vi "BlackJack21.vi"() -> ()   [LabVIEW 2019]
panel:
  out "DRAW":bool
  out "LOSE":bool
  in  "BUST":bool
  out "WIN":bool
  out "DealerCard#5":u16(ring)
  out "CP-Dealer#5":dbl
  out "DealerCard#4":u16(ring)
  out "CP-Dealer#4":dbl
  in  "STAND POS":dbl
  out "SAME CARD DETECTED":bool
  out "DealerCard#3":u16(ring)
  out "CP-Dealer#3":dbl
  out "UserCard#5":u16(ring)
  out "CP-User#5":dbl
  in  "HIT POS":i32
  out "UserCard#4":u16(ring)
  out "CP-User#4":dbl
  out "DealerCard#2":u16(ring)
  out "CP-Dealer#2":dbl
  out "Total Player Point":dbl
  out "Total Dealer Point":dbl
  out "DealerCard#1":u16(ring)
  out "CP-Dealer#1":dbl
  out "UserCard#3":u16(ring)
  out "CP-User#3":dbl
  out "UserCard#2":u16(ring)
  out "CP-User#2":dbl
  in  "RESTART GAME":bool
  in  "STAND":bool
  out "Numeric":i32
  in  "EMERGENCY STOP":bool
  in  "START GAME":bool
  out "CP-User#1":dbl
  out "UserCard#1":u16(ring)
  in  "Hit":bool
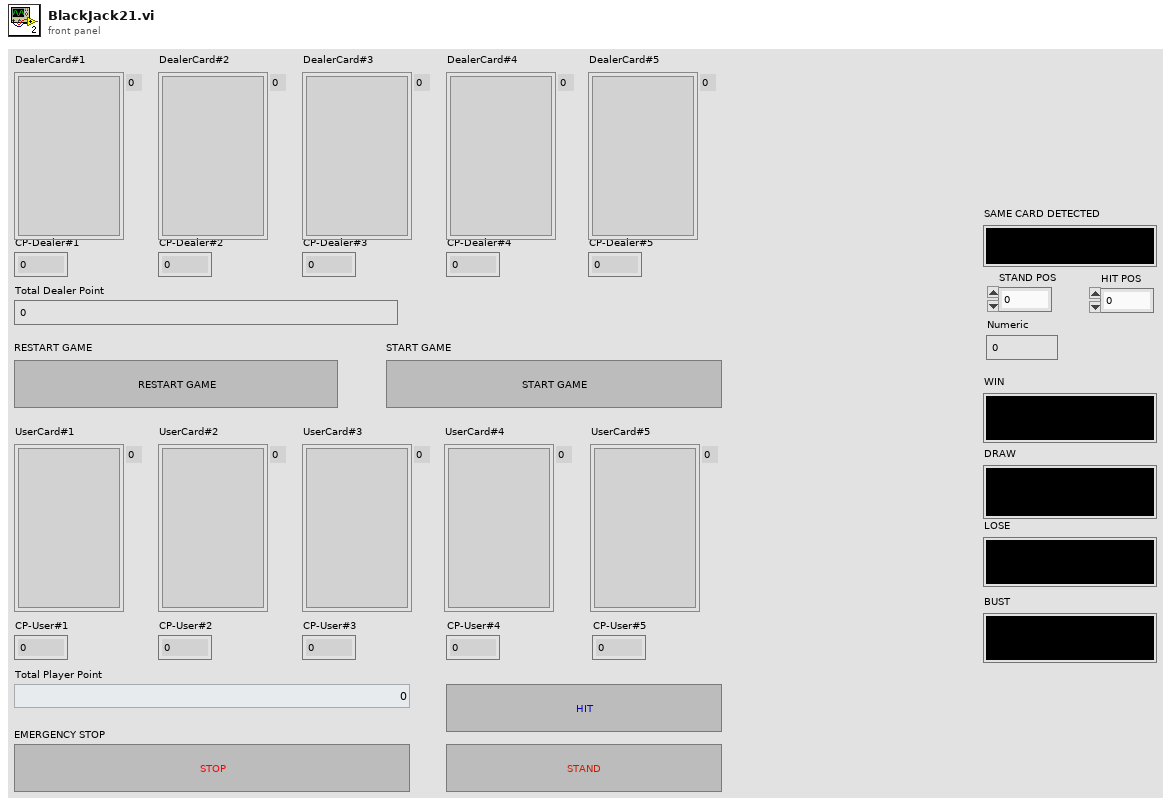
[diagram p1: front panel]
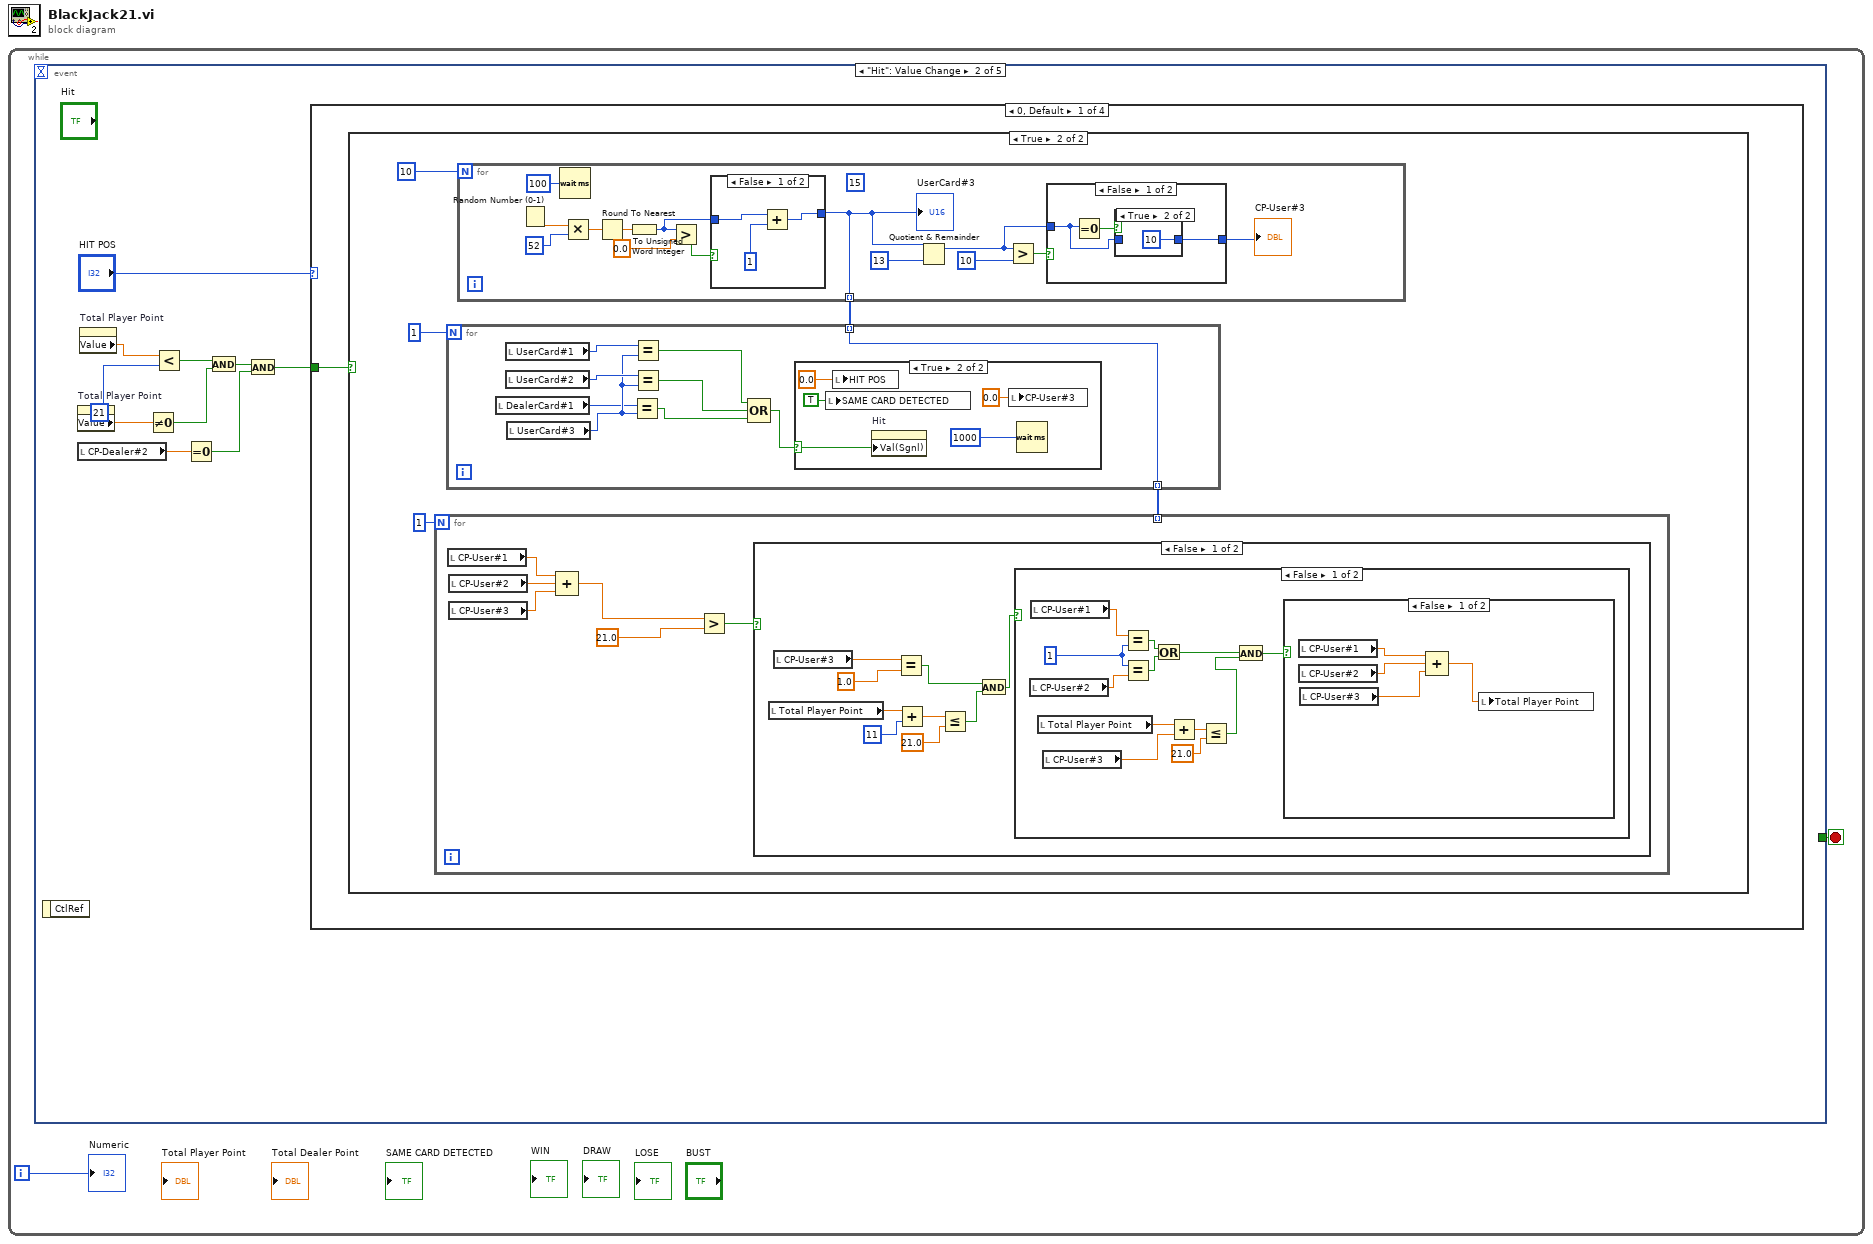
[diagram p0: block diagram]
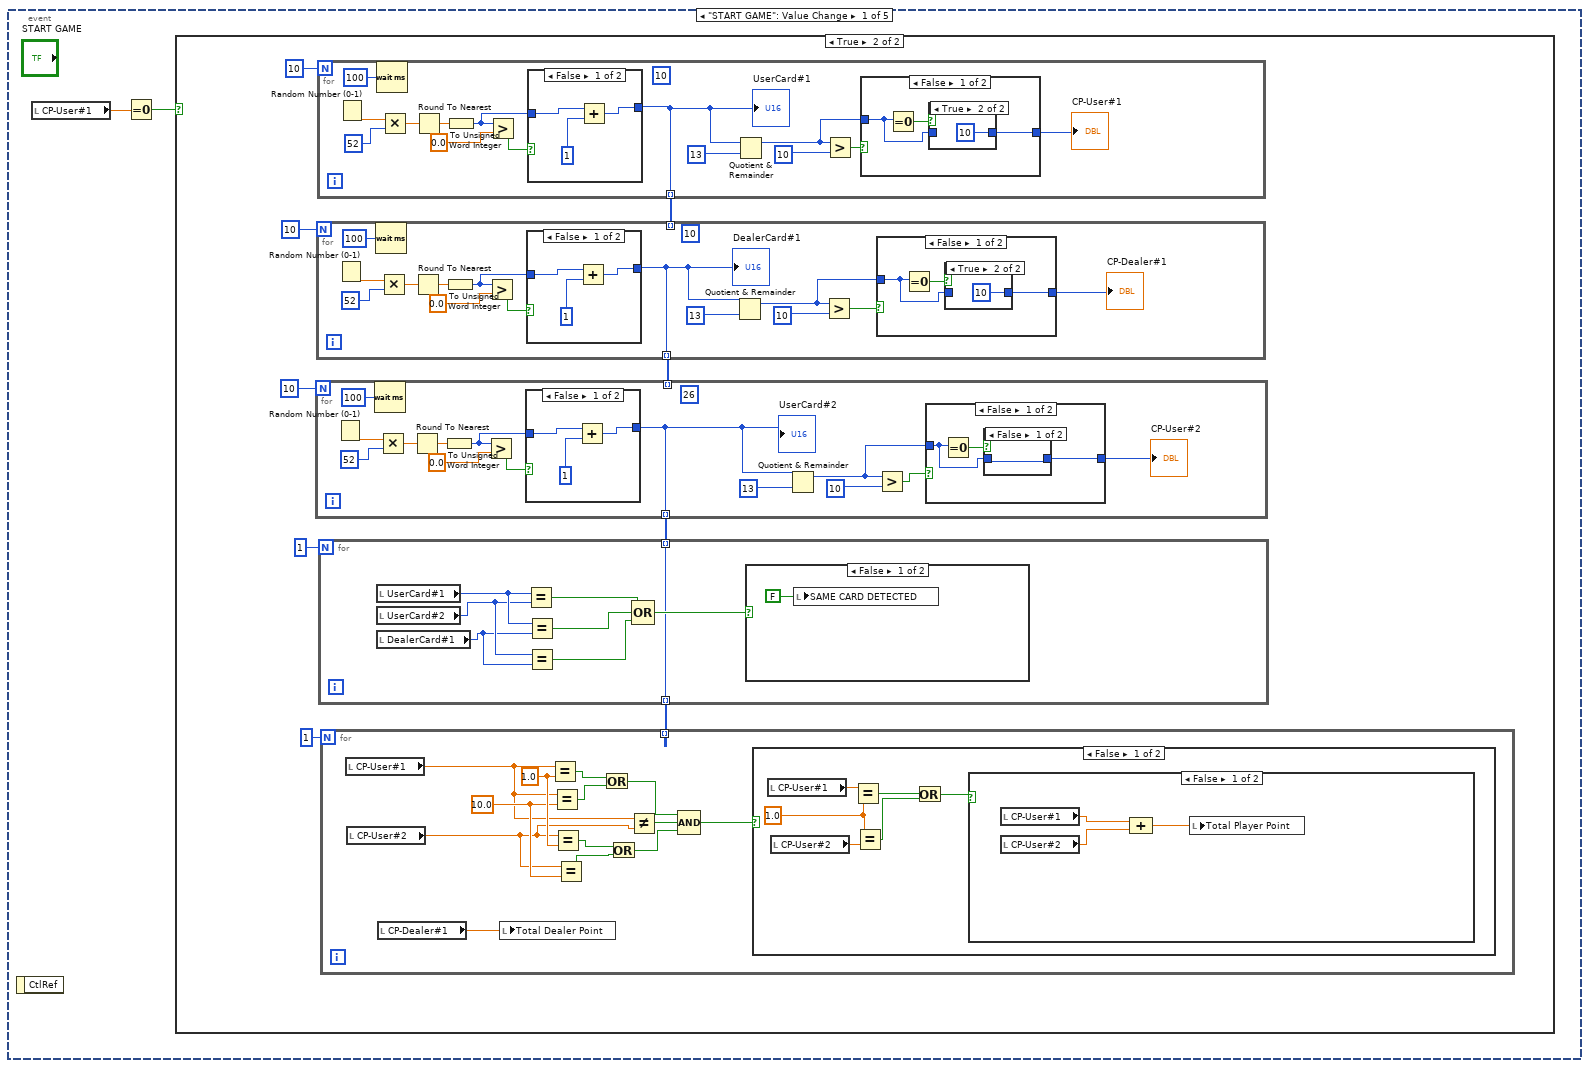
[diagram p2: hidden frame]
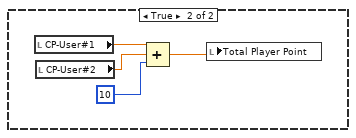
[diagram p4: hidden frame]
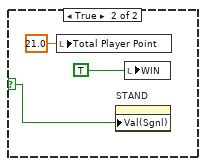
[diagram p5: hidden frame]
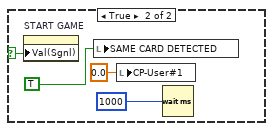
[diagram p6: hidden frame]
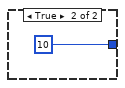
[diagram p8: hidden frame]
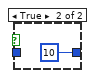
[diagram p10: hidden frame]
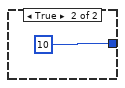
[diagram p11: hidden frame]
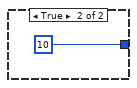
[diagram p14: hidden frame]
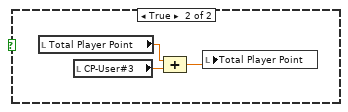
[diagram p17: hidden frame]
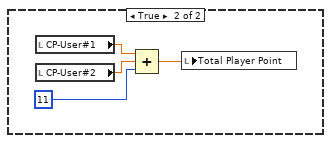
[diagram p18: hidden frame]
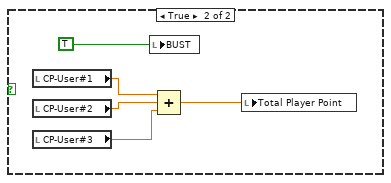
[diagram p19: hidden frame]
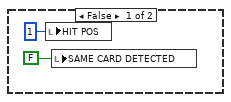
[diagram p20: hidden frame]
diagram:
  n1 = while {
    i -> [w2]
    stop <- w1 stop-if-true
    n2 = event shown="[1] \"Hit\": Value Change" {
      selector: _ -> [_ _ _ _ _]
      dyn-events: _ -> [_ _ _ _ _]
      timeout: _ -> [_ _ _ _ _]
      tunnel: [_ _ _ _ "EMERGENCY STOP"] -> w1
      event "START GAME": Value Change {
        n3 = event-data() -> ()  [unwired: 1 in, 1 out]
        n4 = local read "CP-User#1"() -> (w4:dbl)
        n5 = Equal To 0?(x=w4) -> (x = 0?=w3:bool)
        n6 = case shown="True" w3 {
          frame False {
          }
          frame True {
            n7 = for {
              N: 10 -> [_]
              tunnel: [w104] -> w10 mode=indexing
              (unwired) 10
              n8 = Random Number (0-1)() -> (number: 0 to 1=w117:dbl)
              n9 = Wait (ms)(milliseconds to wait=u32 100) -> ()  [unwired: 1 out]
              n10 = Multiply(x=w117, y=52) -> (x*y=w114:dbl)
              n11 = Round To Nearest(number=w114) -> (nearest integer value=w113:dbl)
              n12 = To Unsigned Word Integer(number=w113) -> (unsigned 16bit integer=w110:u16)
              n13 = Greater?(x=w110, y=0.0) -> (0:w111:bool)
              n14 = case shown="False" w111 {
                tunnel: [w124 w127] -> w104
                tunnel: w110 -> [w126 w127]
                frame False {
                  n15 = Add(x=w126, y=u16 1) -> (x+y=w124:u16)
                }
                frame True {
                }
              }
              "UserCard#1" <- w104
              n16 = Quotient & Remainder(x=w104, y=13) -> (x-y*floor(x/y)=w105:i32)  [unwired: 1 out]
              n17 = Greater?(x=w105, y=10) -> (0:w107:bool)
              n18 = case shown="False" w107 {
                tunnel: [w119 10] -> w106
                tunnel: w105 -> [w118 _]
                frame False {
                  n19 = Equal To 0?(x=w118) -> (x = 0?=w120:bool)
                  n20 = case shown="True" w120 {
                    tunnel: [w121 10] -> w119
                    tunnel: w118 -> [w121 _]
                    frame False {
                    }
                    frame True {
                    }
                  }
                }
                frame True {
                }
              }
              "CP-User#1" <- w106
            }
            n21 = for {
              N: 10 -> [_]
              tunnel: [w56] -> w9 mode=indexing
              tunnel: w10 -> [_] mode=indexing
              (unwired) 10
              n22 = Random Number (0-1)() -> (number: 0 to 1=w69:dbl)
              n23 = Wait (ms)(milliseconds to wait=u32 100) -> ()  [unwired: 1 out]
              n24 = Multiply(x=w69, y=52) -> (x*y=w66:dbl)
              n25 = Round To Nearest(number=w66) -> (nearest integer value=w65:dbl)
              n26 = To Unsigned Word Integer(number=w65) -> (unsigned 16bit integer=w62:u16)
              n27 = Greater?(x=w62, y=0.0) -> (0:w63:bool)
              n28 = case shown="False" w63 {
                tunnel: [w76 w79] -> w56
                tunnel: w62 -> [w78 w79]
                frame False {
                  n29 = Add(x=w78, y=u16 1) -> (x+y=w76:u16)
                }
                frame True {
                }
              }
              "DealerCard#1" <- w56
              n30 = Quotient & Remainder(x=w56, y=13) -> (x-y*floor(x/y)=w58:i32)  [unwired: 1 out]
              n31 = Greater?(x=w58, y=10) -> (0:w59:bool)
              n32 = case shown="False" w59 {
                tunnel: [w71 10] -> w57
                tunnel: w58 -> [w70 _]
                frame False {
                  n33 = Equal To 0?(x=w70) -> (x = 0?=w72:bool)
                  n34 = case shown="True" w72 {
                    tunnel: [w73 10] -> w71
                    tunnel: w70 -> [w73 _]
                    frame False {
                    }
                    frame True {
                    }
                  }
                }
                frame True {
                }
              }
              "CP-Dealer#1" <- w57
            }
            n35 = for {
              N: 10 -> [_]
              tunnel: [w80] -> w7 mode=indexing
              tunnel: w9 -> [_] mode=indexing
              (unwired) 26
              n36 = Random Number (0-1)() -> (number: 0 to 1=w93:dbl)
              n37 = Wait (ms)(milliseconds to wait=u32 100) -> ()  [unwired: 1 out]
              n38 = Multiply(x=w93, y=52) -> (x*y=w90:dbl)
              n39 = Round To Nearest(number=w90) -> (nearest integer value=w89:dbl)
              n40 = To Unsigned Word Integer(number=w89) -> (unsigned 16bit integer=w86:u16)
              n41 = Greater?(x=w86, y=0.0) -> (0:w87:bool)
              n42 = case shown="False" w87 {
                tunnel: [w100 w103] -> w80
                tunnel: w86 -> [w102 w103]
                frame False {
                  n43 = Add(x=w102, y=u16 1) -> (x+y=w100:u16)
                }
                frame True {
                }
              }
              "UserCard#2" <- w80
              n44 = Quotient & Remainder(x=w80, y=13) -> (x-y*floor(x/y)=w81:i32)  [unwired: 1 out]
              n45 = Greater?(x=w81, y=10) -> (0:w83:bool)
              n46 = case shown="False" w83 {
                tunnel: [w95 10] -> w82
                tunnel: w81 -> [w94 _]
                frame False {
                  n47 = Equal To 0?(x=w94) -> (x = 0?=w96:bool)
                  n48 = case shown="False" w96 {
                    tunnel: [w97 10] -> w95
                    tunnel: w94 -> [w97 _]
                    frame False {
                    }
                    frame True {
                    }
                  }
                }
                frame True {
                }
              }
              "CP-User#2" <- w82
            }
            n49 = for {
              N: 1 -> [_]
              tunnel: w7 -> [w43] mode=indexing
              tunnel: [w43] -> w5 mode=indexing
              n50 = local read "UserCard#1"() -> (w46:u16)
              n51 = local read "UserCard#2"() -> (w45:u16)
              n52 = local read "DealerCard#1"() -> (w44:u16)
              n53 = Equal?(x=w46, y=w45) -> (x = y?=w50:bool)
              n54 = Equal?(x=w46, y=w44) -> (x = y?=w49:bool)
              n55 = Equal?(x=w45, y=w44) -> (x = y?=w48:bool)
              n56 = Compound Arithmetic op=OR(w50, w49, w48) -> (w47:bool)
              n57 = case shown="False" w47 {
                selector: w47 -> [_ w55]
                frame False {
                  n58 = local write "SAME CARD DETECTED"(FALSE ("Same Card CASE TRUE!!!!")) -> ()
                }
                frame True {
                  n59 = property on="START GAME" class="Bool (strict)"("Val(Sgnl)"=w55) -> ()  [unwired: 2 in, 2 out]
                  n60 = local write "SAME CARD DETECTED"(TRUE ("Same Card CASE TRUE!!!!")) -> ()
                  n61 = local write "CP-User#1"(0.0 ("CP-User#1")) -> ()
                  n62 = Wait (ms)(milliseconds to wait=u32 1000 ("millisecond timer value")) -> ()  [unwired: 1 out]
                }
              }
            }
            n63 = for {
              N: 1 -> [_]
              tunnel: w5 -> [_] mode=indexing
              w25 = 10.0 ("y")
              w26 = 1.0 ("y")
              n64 = local read "CP-User#1"() -> (w15:dbl)
              n65 = local read "CP-User#2"() -> (w16:dbl)
              n66 = local read "CP-Dealer#1"() -> (w14:dbl)
              n67 = local write "Total Dealer Point"(w14) -> ()
              n68 = Equal?(x=w15, y=w26) -> (x = y?=w23:bool)
              n69 = Equal?(x=w15, y=w25) -> (x = y?=w24:bool)
              n70 = Equal?(x=w16, y=w26) -> (x = y?=w22:bool)
              n71 = Equal?(x=w16, y=w25) -> (x = y?=w21:bool)
              n72 = Or(x=w23, y=w24) -> (x .or. y?=w20:bool)
              n73 = Or(x=w22, y=w21) -> (x .or. y?=w19:bool)
              n74 = Not Equal?(x=w15, y=w16) -> (x != y?=w18:bool)
              n75 = Compound Arithmetic op=AND(w20, w18, w19) -> (w17:bool)
              n76 = case shown="False" w17 {
                selector: w17 -> [_ w41]
                frame False {
                  w31 = 1.0 ("y")
                  n77 = local read "CP-User#1"() -> (w32:dbl)
                  n78 = local read "CP-User#2"() -> (w30:dbl)
                  n79 = Equal?(x=w32, y=w31) -> (x = y?=w29:bool)
                  n80 = Equal?(x=w31, y=w30) -> (x = y?=w28:bool)
                  n81 = Or(x=w29, y=w28) -> (x .or. y?=w27:bool)
                  n82 = case shown="False" w27 {
                    frame False {
                      n83 = local read "CP-User#1"() -> (w34:dbl)
                      n84 = local read "CP-User#2"() -> (w33:dbl)
                      n85 = Compound Arithmetic op=ADD(w34, w33) -> (w35:dbl)
                      n86 = local write "Total Player Point"(w35) -> ()
                    }
                    frame True {
                      n87 = local read "CP-User#1"() -> (w39:dbl)
                      n88 = local read "CP-User#2"() -> (w38:dbl)
                      n89 = Compound Arithmetic op=ADD(w39, w38, 10) -> (w36:dbl)
                      n90 = local write "Total Player Point"(w36) -> ()
                    }
                  }
                }
                frame True {
                  n91 = local write "Total Player Point"(21.0 ("Total Player Point")) -> ()
                  n92 = property on="STAND" class="Bool (strict)"("Val(Sgnl)"=w41) -> ()  [unwired: 2 in, 2 out]
                  n93 = local write "WIN"(TRUE ("WIN")) -> ()
                }
              }
            }
          }
        }
      }
      event "Hit": Value Change {
        n94 = event-data() -> ()  [unwired: 1 in, 1 out]
        n95 = property on="Total Player Point" class="DigNum (strict)"() -> ("Value"=w132:dbl)  [unwired: 2 in, 2 out]
        n96 = local read "CP-Dealer#2"() -> (w134:dbl)
        n97 = property on="Total Player Point" class="DigNum (strict)"() -> ("Value"=w130:dbl)  [unwired: 2 in, 2 out]
        n98 = Not Equal To 0?(x=w132) -> (x != 0?=w133:bool)
        n99 = Less?(x=w130, y=21) -> (x < y?=w131:bool)
        n100 = Equal To 0?(x=w134) -> (x = 0?=w136:bool)
        n101 = And(x=w131, y=w133) -> (x .and. y?=w135:bool)
        n102 = And(x=w135, y=w136) -> (x .and. y?=w128:bool)
        n103 = case shown="0, Default" "HIT POS" {
          tunnel: w128 -> [w138 w227 w321 _]
          frame 0, Default {
            n104 = case shown="True" w138 {
              frame False {
              }
              frame True {
                n105 = for {
                  N: 10 -> [_]
                  tunnel: [w203] -> w141 mode=indexing
                  (unwired) 15
                  n106 = Random Number (0-1)() -> (number: 0 to 1=w216:dbl)
                  n107 = Wait (ms)(milliseconds to wait=u32 100) -> ()  [unwired: 1 out]
                  n108 = Multiply(x=w216, y=52) -> (x*y=w215:dbl)
                  n109 = Round To Nearest(number=w215) -> (nearest integer value=w214:dbl)
                  n110 = To Unsigned Word Integer(number=w214) -> (unsigned 16bit integer=w212:u16)
                  n111 = Greater?(x=w212, y=0.0) -> (0:w213:bool)
                  n112 = case shown="False" w213 {
                    tunnel: [w223 w226] -> w203
                    tunnel: w212 -> [w225 w226]
                    frame False {
                      n113 = Add(x=w225, y=u16 1) -> (x+y=w223:u16)
                    }
                    frame True {
                    }
                  }
                  "UserCard#3" <- w203
                  n114 = Quotient & Remainder(x=w203, y=13) -> (x-y*floor(x/y)=w211:i32)  [unwired: 1 out]
                  n115 = Greater?(x=w211, y=10) -> (0:w210:bool)
                  n116 = case shown="False" w210 {
                    tunnel: [w218 10] -> w209
                    tunnel: w211 -> [w217 _]
                    frame False {
                      n117 = Equal To 0?(x=w217) -> (x = 0?=w219:bool)
                      n118 = case shown="True" w219 {
                        tunnel: [w220 10] -> w218
                        tunnel: w217 -> [w220 _]
                        frame False {
                        }
                        frame True {
                        }
                      }
                    }
                    frame True {
                    }
                  }
                  "CP-User#3" <- w209
                }
                n119 = for {
                  N: 1 -> [_]
                  tunnel: w141 -> [w187] mode=indexing
                  tunnel: [w187] -> w139 mode=indexing
                  n120 = local read "DealerCard#1"() -> (w188:u16)
                  n121 = local read "UserCard#1"() -> (w194:u16)
                  n122 = local read "UserCard#2"() -> (w193:u16)
                  n123 = local read "UserCard#3"() -> (w189:u16)
                  n124 = Equal?(x=w188, y=w189) -> (x = y?=w190:bool)
                  n125 = Equal?(x=w194, y=w189) -> (x = y?=w192:bool)
                  n126 = Equal?(x=w193, y=w189) -> (x = y?=w191:bool)
                  n127 = Compound Arithmetic op=OR(w192, w191, w190) -> (w195:bool)
                  n128 = case shown="True" w195 {
                    selector: w195 -> [_ w201]
                    frame False {
                      n129 = local write "HIT POS"(1 ("HIT POS")) -> ()
                      n130 = local write "SAME CARD DETECTED"(FALSE ("Same Card CASE TRUE!!!!")) -> ()
                    }
                    frame True {
                      n131 = local write "SAME CARD DETECTED"(TRUE ("Same Card CASE TRUE!!!!")) -> ()
                      n132 = local write "HIT POS"(0.0 ("HIT CONTROL")) -> ()
                      n133 = property on="Hit" class="Bool (strict)"("Val(Sgnl)"=w201) -> ()  [unwired: 2 in, 2 out]
                      n134 = local write "CP-User#3"(0.0 ("CP-User#3")) -> ()
                      n135 = Wait (ms)(milliseconds to wait=u32 1000 ("millisecond timer value")) -> ()  [unwired: 1 out]
                    }
                  }
                }
                n136 = for {
                  N: 1 -> [_]
                  tunnel: w139 -> [_] mode=indexing
                  n137 = local read "CP-User#1"() -> (w149:dbl)
                  n138 = local read "CP-User#2"() -> (w148:dbl)
                  n139 = local read "CP-User#3"() -> (w147:dbl)
                  n140 = Compound Arithmetic op=ADD(w149, w148, w147) -> (w146:dbl)
                  n141 = Greater?(x=w146, y=21.0) -> (0:w144:bool)
                  n142 = case shown="False" w144 {
                    frame False {
                      n143 = local read "Total Player Point"() -> (w157:dbl)
                      n144 = local read "CP-User#3"() -> (w153:dbl)
                      n145 = Equal?(x=w153, y=1.0) -> (x = y?=w158:bool)
                      n146 = Add(x=w157, y=11) -> (x+y=w152:dbl)
                      n147 = Less Or Equal?(x=w152, y=21.0) -> (x <= y?=w150:bool)
                      n148 = And(x=w158, y=w150) -> (x .and. y?=w155:bool)
                      n149 = case shown="False" w155 {
                        frame False {
                          w166 = 1
                          n150 = local read "CP-User#2"() -> (w167:dbl)
                          n151 = local read "CP-User#1"() -> (w168:dbl)
                          n152 = local read "Total Player Point"() -> (w165:dbl)
                          n153 = local read "CP-User#3"() -> (w159:dbl)
                          n154 = Equal?(x=w168, y=w166) -> (x = y?=w170:bool)
                          n155 = Equal?(x=w166, y=w167) -> (x = y?=w169:bool)
                          n156 = Or(x=w170, y=w169) -> (x .or. y?=w164:bool)
                          n157 = Add(x=w165, y=w159) -> (x+y=w162:dbl)
                          n158 = Less Or Equal?(x=w162, y=21.0 ("x")) -> (x <= y?=w160:bool)
                          n159 = And(x=w164, y=w160) -> (x .and. y?=w163:bool)
                          n160 = case shown="False" w163 {
                            frame False {
                              n161 = local read "CP-User#1"() -> (w174:dbl)
                              n162 = local read "CP-User#2"() -> (w173:dbl)
                              n163 = local read "CP-User#3"() -> (w172:dbl)
                              n164 = Compound Arithmetic op=ADD(w174, w173, w172) -> (w171:dbl)
                              n165 = local write "Total Player Point"(w171) -> ()
                            }
                            frame True {
                              n166 = local read "Total Player Point"() -> (w175:dbl)
                              n167 = local read "CP-User#3"() -> (w177:dbl)
                              n168 = Compound Arithmetic op=ADD(w175, w177) -> (w176:dbl)
                              n169 = local write "Total Player Point"(w176) -> ()
                            }
                          }
                        }
                        frame True {
                          n170 = local read "CP-User#1"() -> (w181:dbl)
                          n171 = local read "CP-User#2"() -> (w180:dbl)
                          n172 = Compound Arithmetic op=ADD(w181, w180, 11) -> (w178:dbl)
                          n173 = local write "Total Player Point"(w178) -> ()
                        }
                      }
                    }
                    frame True {
                      n174 = local read "CP-User#1"() -> (w185:dbl)
                      n175 = local read "CP-User#2"() -> (w184:dbl)
                      n176 = local read "CP-User#3"() -> (w183:dbl)
                      n177 = local write "BUST"(TRUE ("WINNER INDICATOR [DEALER]")) -> ()
                      n178 = Compound Arithmetic op=ADD(w185, w184, w183) -> (w182:dbl)
                      n179 = local write "Total Player Point"(w182) -> ()
                    }
                  }
                }
              }
            }
          }
          frame 1 {
            n180 = case shown="True" w227 {
              frame False {
              }
              frame True {
                n181 = for {
                  N: 10 -> [_]
                  tunnel: [w297] -> w230 mode=indexing
                  (unwired) 28
                  n182 = Random Number (0-1)() -> (number: 0 to 1=w310:dbl)
                  n183 = Wait (ms)(milliseconds to wait=u32 100) -> ()  [unwired: 1 out]
                  n184 = Multiply(x=w310, y=52) -> (x*y=w307:dbl)
                  n185 = Round To Nearest(number=w307) -> (nearest integer value=w306:dbl)
                  n186 = To Unsigned Word Integer(number=w306) -> (unsigned 16bit integer=w303:u16)
                  n187 = Greater?(x=w303, y=0.0) -> (0:w304:bool)
                  n188 = case shown="False" w304 {
                    tunnel: [w317 w320] -> w297
                    tunnel: w303 -> [w319 w320]
                    frame False {
                      n189 = Add(x=w319, y=u16 1) -> (x+y=w317:u16)
                    }
                    frame True {
                    }
                  }
                  "UserCard#4" <- w297
                  n190 = Quotient & Remainder(x=w297, y=13) -> (x-y*floor(x/y)=w300:i32)  [unwired: 1 out]
                  n191 = Greater?(x=w300, y=10) -> (0:w299:bool)
                  n192 = case shown="False" w299 {
                    tunnel: [w312 10] -> w298
                    tunnel: w300 -> [w311 _]
                    frame False {
                      n193 = Equal To 0?(x=w311) -> (x = 0?=w313:bool)
                      n194 = case shown="True" w313 {
                        tunnel: [w314 10] -> w312
                        tunnel: w311 -> [w314 _]
                        frame False {
                        }
                        frame True {
                        }
                      }
                    }
                    frame True {
                    }
                  }
                  "CP-User#4" <- w298
                }
                n195 = for {
                  N: 1 -> [_]
                  tunnel: w230 -> [w282] mode=indexing
                  tunnel: [w282] -> w229 mode=indexing
                  n196 = local read "DealerCard#1"() -> (w289:u16)
                  n197 = local read "UserCard#4"() -> (w288:u16)
                  n198 = local read "UserCard#1"() -> (w285:u16)
                  n199 = local read "UserCard#2"() -> (w286:u16)
                  n200 = local read "UserCard#3"() -> (w287:u16)
                  n201 = formula code="if(U4==U1)\nx = 0;\nelse if(U4==U2)\nx = 0;\nelse if (U4==U3)\nx = 0;\nelse if (U4==D1)\nx = 0;\nelse\nx = 1;"("U1"=w285, "U2"=w286, "U3"=w287, "U4"=w288, "D1"=w289) -> ("x"=w284:dbl)
                  n202 = Equal To 0?(x=w284) -> (x = 0?=w283:bool)
                  n203 = case shown="True" w283 {
                    selector: w283 -> [_ w294]
                    frame False {
                      n204 = local write "HIT POS"(2) -> ()
                      n205 = local write "SAME CARD DETECTED"(FALSE) -> ()
                    }
                    frame True {
                      n206 = local write "HIT POS"(1 ("HIT POS")) -> ()
                      n207 = local write "SAME CARD DETECTED"(TRUE) -> ()
                      n208 = property on="Hit" class="Bool (strict)"("Val(Sgnl)"=w294) -> ()  [unwired: 2 in, 2 out]
                      n209 = local write "CP-User#4"(0.0 ("CP-User#4")) -> ()
                      n210 = Wait (ms)(milliseconds to wait=u32 1000 ("millisecond timer value")) -> ()  [unwired: 1 out]
                    }
                  }
                }
                n211 = for {
                  N: 1 -> [_]
                  tunnel: w229 -> [_] mode=indexing
                  n212 = local read "CP-User#2"() -> (w238:dbl)
                  n213 = local read "CP-User#3"() -> (w237:dbl)
                  n214 = local read "CP-User#1"() -> (w239:dbl)
                  n215 = local read "CP-User#4"() -> (w236:dbl)
                  n216 = Compound Arithmetic op=ADD(w239, w238, w237, w236) -> (w234:dbl)
                  n217 = Greater?(x=w234, y=21.0) -> (0:w235:bool)
                  n218 = case shown="False" w235 {
                    frame False {
                      n219 = local read "Total Player Point"() -> (w246:dbl)
                      n220 = local read "CP-User#4"() -> (w248:dbl)
                      n221 = Equal?(x=w248, y=1.0) -> (x = y?=w242:bool)
                      n222 = Add(x=w246, y=11.0 ("x")) -> (x+y=w244:dbl)
                      n223 = Less Or Equal?(x=w244, y=21) -> (x <= y?=w241:bool)
                      n224 = And(x=w242, y=w241) -> (x .and. y?=w240:bool)
                      n225 = case shown="False" w240 {
                        frame False {
                          w260 = 1
                          n226 = local read "Total Player Point"() -> (w255:dbl)
                          n227 = local read "CP-User#3"() -> (w262:dbl)
                          n228 = local read "CP-User#1"() -> (w259:dbl)
                          n229 = local read "CP-User#2"() -> (w261:dbl)
                          n230 = local read "CP-User#4"() -> (w254:dbl)
                          n231 = Equal?(x=w259, y=w260) -> (x = y?=w258:bool)
                          n232 = Equal?(x=w261, y=w260) -> (x = y?=w257:bool)
                          n233 = Equal?(x=w260, y=w262) -> (x = y?=w256:bool)
                          n234 = Add(x=w255, y=w254) -> (x+y=w253:dbl)
                          n235 = Compound Arithmetic op=OR(w258, w257, w256) -> (w251:bool)
                          n236 = Less Or Equal?(x=w253, y=21.0) -> (x <= y?=w250:bool)
                          n237 = And(x=w251, y=w250) -> (x .and. y?=w249:bool)
                          n238 = case shown="True" w249 {
                            frame False {
                              n239 = local read "CP-User#1"() -> (w263:dbl)
                              n240 = local read "CP-User#2"() -> (w264:dbl)
                              n241 = local read "CP-User#3"() -> (w265:dbl)
                              n242 = local read "CP-User#4"() -> (w266:dbl)
                              n243 = Compound Arithmetic op=ADD(w263, w264, w265, w266) -> (w267:dbl)
                              n244 = local write "Total Player Point"(w267) -> ()
                            }
                            frame True {
                              n245 = local read "Total Player Point"() -> (w270:dbl)
                              n246 = local read "CP-User#4"() -> (w269:dbl)
                              n247 = Add(x=w270, y=w269) -> (x+y=w268:dbl)
                              n248 = local write "Total Player Point"(w268) -> ()
                            }
                          }
                        }
                        frame True {
                          n249 = local read "CP-User#3"() -> (w273:dbl)
                          n250 = local read "CP-User#2"() -> (w274:dbl)
                          n251 = local read "CP-User#1"() -> (w275:dbl)
                          n252 = Compound Arithmetic op=ADD(w275, w274, w273, 11) -> (w271:dbl)
                          n253 = local write "Total Player Point"(w271) -> ()
                        }
                      }
                    }
                    frame True {
                      n254 = local read "CP-User#1"() -> (w280:dbl)
                      n255 = local read "CP-User#2"() -> (w279:dbl)
                      n256 = local read "CP-User#3"() -> (w278:dbl)
                      n257 = local read "CP-User#4"() -> (w277:dbl)
                      n258 = local write "BUST"(TRUE ("WINNER INDICATOR [DEALER]")) -> ()
                      n259 = Compound Arithmetic op=ADD(w280, w279, w278, w277) -> (w276:dbl)
                      n260 = local write "Total Player Point"(w276) -> ()
                    }
                  }
                }
              }
            }
          }
          frame 2 {
            n261 = case shown="True" w321 {
              frame False {
              }
              frame True {
                n262 = for {
                  N: 10 -> [_]
                  tunnel: [w402] -> w324 mode=indexing
                  (unwired) 42
                  n263 = Random Number (0-1)() -> (number: 0 to 1=w415:dbl)
                  n264 = Wait (ms)(milliseconds to wait=u32 100) -> ()  [unwired: 1 out]
                  n265 = Multiply(x=w415, y=52) -> (x*y=w412:dbl)
                  n266 = Round To Nearest(number=w412) -> (nearest integer value=w411:dbl)
                  n267 = To Unsigned Word Integer(number=w411) -> (unsigned 16bit integer=w408:u16)
                  n268 = Greater?(x=w408, y=0.0) -> (0:w409:bool)
                  n269 = case shown="False" w409 {
                    tunnel: [w422 w425] -> w402
                    tunnel: w408 -> [w424 w425]
                    frame False {
                      n270 = Add(x=w424, y=u16 1) -> (x+y=w422:u16)
                    }
                    frame True {
                    }
                  }
                  "UserCard#5" <- w402
                  n271 = Quotient & Remainder(x=w402, y=13) -> (x-y*floor(x/y)=w405:i32)  [unwired: 1 out]
                  n272 = Greater?(x=w405, y=10) -> (0:w404:bool)
                  n273 = case shown="False" w404 {
                    tunnel: [w417 10] -> w403
                    tunnel: w405 -> [w416 _]
                    frame False {
                      n274 = Equal To 0?(x=w416) -> (x = 0?=w418:bool)
                      n275 = case shown="True" w418 {
                        tunnel: [w419 10] -> w417
                        tunnel: w416 -> [w419 _]
                        frame False {
                        }
                        frame True {
                        }
                      }
                    }
                    frame True {
                    }
                  }
                  "CP-User#5" <- w403
                }
                n276 = for {
                  N: 1 -> [_]
                  tunnel: w324 -> [w382] mode=indexing
                  tunnel: [w382] -> w323 mode=indexing
                  n277 = local read "UserCard#1"() -> (w389:u16)
                  n278 = local read "UserCard#2"() -> (w390:u16)
                  n279 = local read "UserCard#3"() -> (w391:u16)
                  n280 = local read "UserCard#4"() -> (w392:u16)
                  n281 = local read "DealerCard#1"() -> (w393:u16)
                  n282 = local read "UserCard#5"() -> (w394:u16)
                  n283 = Equal?(x=w389, y=w394) -> (x = y?=w388:bool)
                  n284 = Equal?(x=w390, y=w394) -> (x = y?=w387:bool)
                  n285 = Equal?(x=w391, y=w394) -> (x = y?=w386:bool)
                  n286 = Equal?(x=w392, y=w394) -> (x = y?=w385:bool)
                  n287 = Equal?(x=w393, y=w394) -> (x = y?=w384:bool)
                  n288 = Compound Arithmetic op=OR(w388, w387, w386, w385, w384) -> (w383:bool)
                  n289 = case shown="True" w383 {
                    selector: w383 -> [_ w400]
                    frame False {
                      n290 = local write "HIT POS"(3 ("HIT POS")) -> ()
                      n291 = local write "SAME CARD DETECTED"(FALSE ("SAME CARD DETECTED")) -> ()
                    }
                    frame True {
                      n292 = property on="Hit" class="Bool (strict)"("Val(Sgnl)"=w400) -> ()  [unwired: 2 in, 2 out]
                      n293 = local write "HIT POS"(2) -> ()
                      n294 = local write "SAME CARD DETECTED"(TRUE) -> ()
                      n295 = Wait (ms)(milliseconds to wait=u32 1000 ("millisecond timer value")) -> ()  [unwired: 1 out]
                      n296 = local write "CP-User#5"(0.0 ("CP-User#5")) -> ()
                    }
                  }
                }
                n297 = for {
                  N: 1 -> [_]
                  tunnel: w323 -> [_] mode=indexing
                  n298 = local read "CP-User#3"() -> (w332:dbl)
                  n299 = local read "CP-User#4"() -> (w333:dbl)
                  n300 = local read "CP-User#1"() -> (w330:dbl)
                  n301 = local read "CP-User#2"() -> (w331:dbl)
                  n302 = local read "CP-User#5"() -> (w334:dbl)
                  n303 = Compound Arithmetic op=ADD(w330, w331, w332, w333, w334) -> (w328:dbl)
                  n304 = Greater?(x=w328, y=21.0) -> (0:w329:bool)
                  n305 = case shown="False" w329 {
                    frame False {
                      n306 = local read "Total Player Point"() -> (w341:dbl)
                      n307 = local read "CP-User#5"() -> (w343:dbl)
                      n308 = Equal?(x=w343, y=1.0) -> (x = y?=w335:bool)
                      n309 = Add(x=w341, y=11.0) -> (x+y=w339:dbl)
                      n310 = Less Or Equal?(x=w339, y=21.0) -> (x <= y?=w337:bool)
                      n311 = And(x=w335, y=w337) -> (x .and. y?=w336:bool)
                      n312 = case shown="True" w336 {
                        frame False {
                          w359 = 1
                          n313 = local read "CP-User#1"() -> (w358:dbl)
                          n314 = local read "CP-User#2"() -> (w357:dbl)
                          n315 = local read "CP-User#3"() -> (w356:dbl)
                          n316 = local read "CP-User#4"() -> (w355:dbl)
                          n317 = local read "Total Player Point"() -> (w350:dbl)
                          n318 = local read "CP-User#5"() -> (w349:dbl)
                          n319 = Equal?(x=w358, y=w359) -> (x = y?=w354:bool)
                          n320 = Equal?(x=w357, y=w359) -> (x = y?=w353:bool)
                          n321 = Equal?(x=w356, y=w359) -> (x = y?=w352:bool)
                          n322 = Equal?(x=w355, y=w359) -> (x = y?=w351:bool)
                          n323 = Add(x=w350, y=w349) -> (x+y=w348:dbl)
                          n324 = Compound Arithmetic op=OR(w354, w353, w352, w351) -> (w345:bool)
                          n325 = Less Or Equal?(x=w348, y=21.0) -> (x <= y?=w344:bool)
                          n326 = And(x=w345, y=w344) -> (x .and. y?=w346:bool)
                          n327 = case shown="True" w346 {
                            frame False {
                              n328 = local read "CP-User#1"() -> (w365:dbl)
                              n329 = local read "CP-User#2"() -> (w364:dbl)
                              n330 = local read "CP-User#4"() -> (w362:dbl)
                              n331 = local read "CP-User#3"() -> (w363:dbl)
                              n332 = local read "CP-User#5"() -> (w361:dbl)
                              n333 = Compound Arithmetic op=ADD(w365, w364, w363, w362, w361) -> (w360:dbl)
                              n334 = local write "Total Player Point"(w360) -> ()
                            }
                            frame True {
                              n335 = local read "Total Player Point"() -> (w367:dbl)
                              n336 = local read "CP-User#5"() -> (w368:dbl)
                              n337 = Add(x=w367, y=w368) -> (x+y=w366:dbl)
                              n338 = local write "Total Player Point"(w366) -> ()
                            }
                          }
                        }
                        frame True {
                          n339 = local read "CP-User#3"() -> (w372:dbl)
                          n340 = local read "CP-User#4"() -> (w371:dbl)
                          n341 = local read "CP-User#1"() -> (w374:dbl)
                          n342 = local read "CP-User#2"() -> (w373:dbl)
                          n343 = Compound Arithmetic op=ADD(w374, w373, w372, w371, 11) -> (w369:dbl)
                          n344 = local write "Total Player Point"(w369) -> ()
                        }
                      }
                    }
                    frame True {
                      n345 = local read "CP-User#1"() -> (w379:dbl)
                      n346 = local read "CP-User#2"() -> (w380:dbl)
                      n347 = local read "CP-User#3"() -> (w378:dbl)
                      n348 = local read "CP-User#4"() -> (w377:dbl)
                      n349 = local read "CP-User#5"() -> (w376:dbl)
                      n350 = local write "BUST"(TRUE ("WINNER INDICATOR [DEALER]")) -> ()
                      n351 = Compound Arithmetic op=ADD(w379, w380, w378, w377, w376) -> (w375:dbl)
                      n352 = local write "Total Player Point"(w375) -> ()
                    }
                  }
                }
              }
            }
          }
          frame 3 {
          }
        }
      }
      event "STAND": Value Change {
        n353 = event-data() -> ()  [unwired: 1 in, 1 out]
        n354 = case shown="3" "STAND POS" {
          frame 0, Default {
            n355 = local read "Total Player Point"() -> (w428:dbl)
            n356 = local read "CP-Dealer#2"() -> (w432:dbl)
            n357 = Not Equal To 0?(x=w428) -> (x != 0?=w431:bool)
            n358 = Less Or Equal?(x=w428, y=21) -> (x <= y?=w427:bool)
            n359 = Equal To 0?(x=w432) -> (x = 0?=w434:bool)
            n360 = And(x=w431, y=w427) -> (x .and. y?=w433:bool)
            n361 = And(x=w433, y=w434) -> (x .and. y?=w430:bool)
            n362 = case shown="True" w430 {
              frame False {
              }
              frame True {
                n363 = for {
                  N: 10 -> [_]
                  tunnel: [w519] -> w437 mode=indexing
                  (unwired) 8
                  n364 = Random Number (0-1)() -> (number: 0 to 1=w532:dbl)
                  n365 = Wait (ms)(milliseconds to wait=u32 100) -> ()  [unwired: 1 out]
                  n366 = Multiply(x=w532, y=52) -> (x*y=w529:dbl)
                  n367 = Round To Nearest(number=w529) -> (nearest integer value=w528:dbl)
                  n368 = To Unsigned Word Integer(number=w528) -> (unsigned 16bit integer=w525:u16)
                  n369 = Greater?(x=w525, y=0.0) -> (0:w526:bool)
                  n370 = case shown="False" w526 {
                    tunnel: [w539 w542] -> w519
                    tunnel: w525 -> [w541 w542]
                    frame False {
                      n371 = Add(x=w541, y=u16 1) -> (x+y=w539:u16)
                    }
                    frame True {
                    }
                  }
                  "DealerCard#2" <- w519
                  n372 = Quotient & Remainder(x=w519, y=13) -> (x-y*floor(x/y)=w522:i32)  [unwired: 1 out]
                  n373 = Greater?(x=w522, y=10) -> (0:w521:bool)
                  n374 = case shown="False" w521 {
                    tunnel: [w534 10] -> w520
                    tunnel: w522 -> [w533 _]
                    frame False {
                      n375 = Equal To 0?(x=w533) -> (x = 0?=w535:bool)
                      n376 = case shown="True" w535 {
                        tunnel: [w536 10] -> w534
                        tunnel: w533 -> [w536 _]
                        frame False {
                        }
                        frame True {
                        }
                      }
                    }
                    frame True {
                    }
                  }
                  "CP-Dealer#2" <- w520
                }
                n377 = for {
                  N: 1 -> [_]
                  tunnel: w437 -> [w497] mode=indexing
                  tunnel: [w497] -> w435 mode=indexing
                  n378 = local read "UserCard#2"() -> (w510:u16)
                  n379 = local read "UserCard#3"() -> (w509:u16)
                  n380 = local read "UserCard#4"() -> (w508:u16)
                  n381 = local read "DealerCard#2"() -> (w505:u16)
                  n382 = local read "UserCard#1"() -> (w511:u16)
                  n383 = local read "UserCard#5"() -> (w507:u16)
                  n384 = local read "DealerCard#1"() -> (w506:u16)
                  n385 = Equal?(x=w511, y=w505) -> (x = y?=w504:bool)
                  n386 = Equal?(x=w510, y=w505) -> (x = y?=w503:bool)
                  n387 = Equal?(x=w509, y=w505) -> (x = y?=w502:bool)
                  n388 = Equal?(x=w508, y=w505) -> (x = y?=w501:bool)
                  n389 = Equal?(x=w507, y=w505) -> (x = y?=w500:bool)
                  n390 = Equal?(x=w506, y=w505) -> (x = y?=w499:bool)
                  n391 = Compound Arithmetic op=OR(w504, w503, w502, w501, w500, w499) -> (w498:bool)
                  n392 = case shown="False" w498 {
                    selector: w498 -> [_ w514]
                    frame False {
                      n393 = local write "STAND POS"(1.0 ("STAND POS")) -> ()
                      n394 = local write "SAME CARD DETECTED"(FALSE ("SAME CARD DETECTED")) -> ()
                    }
                    frame True {
                      n395 = local write "STAND POS"(0.0 ("STAND POS")) -> ()
                      n396 = local write "SAME CARD DETECTED"(TRUE ("SAME CARD DETECTED")) -> ()
                      n397 = property on="STAND" class="Bool (strict)"("Val(Sgnl)"=w514) -> ()  [unwired: 2 in, 2 out]
                      n398 = local write "CP-Dealer#2"(0.0 ("CP-Dealer#2")) -> ()
                      n399 = Wait (ms)(milliseconds to wait=u32 1000) -> ()  [unwired: 1 out]
                    }
                  }
                }
                n400 = for {
                  N: 1 -> [_]
                  tunnel: w435 -> [_] mode=indexing
                  w440 = 1.0 ("y")
                  w443 = 10.0 ("y")
                  n401 = local read "CP-Dealer#1"() -> (w442:dbl)
                  n402 = local read "CP-Dealer#2"() -> (w441:dbl)
                  n403 = Equal?(x=w442, y=w440) -> (x = y?=w450:bool)
                  n404 = Not Equal?(x=w442, y=w441) -> (x != y?=w445:bool)
                  n405 = Equal?(x=w441, y=w440) -> (x = y?=w449:bool)
                  n406 = Equal?(x=w441, y=w443) -> (x = y?=w448:bool)
                  n407 = Equal?(x=w442, y=w443) -> (x = y?=w451:bool)
                  n408 = Or(x=w450, y=w451) -> (x .or. y?=w447:bool)
                  n409 = Or(x=w449, y=w448) -> (x .or. y?=w446:bool)
                  n410 = Compound Arithmetic op=AND(w447, w445, w446) -> (w444:bool)
                  n411 = case shown="False" w444 {
                    frame False {
                      w462 = 1
                      n412 = local read "CP-Dealer#2"() -> (w458:dbl)
                      n413 = local read "CP-Dealer#1"() -> (w459:dbl)
                      n414 = local read "CP-Dealer#1"() -> (w456:dbl)
                      n415 = local read "CP-Dealer#2"() -> (w455:dbl)
                      n416 = Equal?(x=w459, y=w462) -> (x = y?=w463:bool)
                      n417 = Equal?(x=w462, y=w458) -> (x = y?=w464:bool)
                      n418 = Or(x=w463, y=w464) -> (x .or. y?=w461:bool)
                      n419 = Compound Arithmetic op=ADD(w456, w455, 10.0 ("value")) -> (w454:dbl)
                      n420 = Not Equal?(x=w454, y=17.0) -> (x != y?=w452:bool)
                      n421 = And(x=w461, y=w452) -> (x .and. y?=w460:bool)
                      n422 = case shown="False" w460 {
                        selector: w460 -> [w468 w477]
                        frame False {
                          n423 = local read "Total Player Point"() -> (w467:dbl)
                          n424 = property on="STAND" class="Bool (strict)"("Val(Sgnl)"=w468) -> ()  [unwired: 2 in, 2 out]
                          n425 = local read "CP-Dealer#1"() -> (w470:dbl)
                          n426 = local read "CP-Dealer#2"() -> (w469:dbl)
                          n427 = Add(x=w470, y=w469) -> (x+y=w466:dbl)
                          n428 = formula code="if(UP > DP && DP > 16)\nWIN = 0;\nelse if(UP < DP && DP > 16)\nWIN = 1;\nelse if(UP == DP && DP > 16) \nWIN = 2;\nelse\nWIN = 3;"("UP"=w467, "DP"=w466) -> ("WIN"=w465:dbl)
                          n429 = local write "Total Dealer Point"(w466) -> ()
                          n430 = case shown="3" w465 {
                            frame 0, Default {
                              n431 = local write "WIN"(TRUE ("WIN")) -> ()
                            }
                            frame 1 {
                              n432 = local write "LOSE"(TRUE ("LOSE")) -> ()
                            }
                            frame 2 {
                              n433 = local write "DRAW"(TRUE ("DRAW")) -> ()
                            }
                            frame 3 {
                              n434 = local write "DRAW"(FALSE ("DRAW")) -> ()
                              n435 = local write "WIN"(FALSE ("WIN")) -> ()
                              n436 = local write "LOSE"(FALSE ("LOSE")) -> ()
                            }
                          }
                        }
                        frame True {
                          n437 = local read "Total Player Point"() -> (w480:dbl)
                          n438 = local read "CP-Dealer#1"() -> (w483:dbl)
                          n439 = local read "CP-Dealer#2"() -> (w482:dbl)
                          n440 = property on="STAND" class="Bool (strict)"("Val(Sgnl)"=w477) -> ()  [unwired: 2 in, 2 out]
                          n441 = Compound Arithmetic op=ADD(w483, w482, 10.0 ("value")) -> (w481:dbl)
                          n442 = formula code="if (UP > DP && DP > 16)\nWIN = 1;\nelse if (UP < DP && DP > 16)\nWIN = 1;\nelse if (UP = DP && DP > 16)\nWIN = 2;\nelse\nWIN = 3;"("DP"=w481, "UP"=w480) -> ("WIN"=w479:dbl)
                          n443 = local write "Total Dealer Point"(w481) -> ()
                          n444 = case shown="1" w479 {
                            frame 0, Default {
                              n445 = local write "WIN"(TRUE) -> ()
                            }
                            frame 1 {
                              n446 = local write "LOSE"(TRUE ("LOSE")) -> ()
                            }
                            frame 2 {
                              n447 = local write "DRAW"(TRUE ("DRAW")) -> ()
                            }
                            frame 3 {
                              n448 = local write "DRAW"(FALSE ("DRAW")) -> ()
                              n449 = local write "LOSE"(FALSE ("LOSE")) -> ()
                              n450 = local write "WIN"(FALSE ("WIN")) -> ()
                            }
                          }
                        }
                      }
                    }
                    frame True {
                      w492 = 21
                      n451 = local read "Total Player Point"() -> (w491:dbl)
                      n452 = local write "Total Dealer Point"(w492) -> ()
                      n453 = formula code="if(UP > DP)\nWINNER = 0;\nelse if (UP < DP)\nWINNER = 1;\nelse if (UP == DP)\nWINNER = 2;"("DP"=w492, "UP"=w491) -> ("WINNER"=w490:dbl)
                      n454 = case shown="0, Default" w490 {
                        frame 0, Default {
                          n455 = local write "WIN"(TRUE ("WIN")) -> ()
                        }
                        frame 1 {
                          n456 = local write "LOSE"(TRUE ("LOSE")) -> ()
                        }
                        frame 2 {
                          n457 = local write "WIN"(FALSE ("WIN")) -> ()
                          n458 = local write "DRAW"(TRUE ("DRAW")) -> ()
                        }
                      }
                    }
                  }
                }
              }
            }
          }
          frame 1 {
            n459 = local read "Total Dealer Point"() -> (w543:dbl)
            n460 = Less?(x=w543, y=17) -> (x < y?=w544:bool)
            n461 = case shown="True" w544 {
              frame False {
              }
              frame True {
                n462 = for {
                  N: 10 -> [_]
                  tunnel: [w628] -> w548 mode=indexing
                  (unwired) 40
                  n463 = Random Number (0-1)() -> (number: 0 to 1=w641:dbl)
                  n464 = Wait (ms)(milliseconds to wait=u32 100) -> ()  [unwired: 1 out]
                  n465 = Multiply(x=w641, y=52) -> (x*y=w638:dbl)
                  n466 = Round To Nearest(number=w638) -> (nearest integer value=w637:dbl)
                  n467 = To Unsigned Word Integer(number=w637) -> (unsigned 16bit integer=w634:u16)
                  n468 = Greater?(x=w634, y=0.0) -> (0:w635:bool)
                  n469 = case shown="True" w635 {
                    tunnel: [w648 w651] -> w628
                    tunnel: w634 -> [w650 w651]
                    frame False {
                      n470 = Add(x=w650, y=u16 1) -> (x+y=w648:u16)
                    }
                    frame True {
                    }
                  }
                  "DealerCard#3" <- w628
                  n471 = Quotient & Remainder(x=w628, y=13) -> (x-y*floor(x/y)=w631:i32)  [unwired: 1 out]
                  n472 = Greater?(x=w631, y=10) -> (0:w630:bool)
                  n473 = case shown="False" w630 {
                    tunnel: [w643 10] -> w629
                    tunnel: w631 -> [w642 _]
                    frame False {
                      n474 = Equal To 0?(x=w642) -> (x = 0?=w644:bool)
                      n475 = case shown="True" w644 {
                        tunnel: [w645 10] -> w643
                        tunnel: w642 -> [w645 _]
                        frame False {
                        }
                        frame True {
                        }
                      }
                    }
                    frame True {
                    }
                  }
                  "CP-Dealer#3" <- w629
                }
                n476 = for {
                  N: 1 -> [_]
                  tunnel: w548 -> [w604] mode=indexing
                  tunnel: [w604] -> w546 mode=indexing
                  n477 = local read "UserCard#1"() -> (w620:u16)
                  n478 = local read "UserCard#2"() -> (w619:u16)
                  n479 = local read "UserCard#3"() -> (w618:u16)
                  n480 = local read "UserCard#4"() -> (w617:u16)
                  n481 = local read "UserCard#5"() -> (w616:u16)
                  n482 = local read "DealerCard#1"() -> (w615:u16)
                  n483 = local read "DealerCard#2"() -> (w614:u16)
                  n484 = local read "DealerCard#3"() -> (w613:u16)
                  n485 = Equal?(x=w620, y=w613) -> (x = y?=w612:bool)
                  n486 = Equal?(x=w619, y=w613) -> (x = y?=w611:bool)
                  n487 = Equal?(x=w618, y=w613) -> (x = y?=w610:bool)
                  n488 = Equal?(x=w617, y=w613) -> (x = y?=w609:bool)
                  n489 = Equal?(x=w616, y=w613) -> (x = y?=w608:bool)
                  n490 = Equal?(x=w615, y=w613) -> (x = y?=w607:bool)
                  n491 = Equal?(x=w614, y=w613) -> (x = y?=w606:bool)
                  n492 = Compound Arithmetic op=OR(w612, w611, w610, w609, w608, w607, w606) -> (w605:bool)
                  n493 = case shown="True" w605 {
                    selector: w605 -> [_ w625]
                    frame False {
                      n494 = local write "SAME CARD DETECTED"(FALSE ("SAME CARD DETECTED")) -> ()
                      n495 = local write "STAND POS"(2.0 ("STAND POS")) -> ()
                    }
                    frame True {
                      n496 = local write "STAND POS"(1.0 ("STAND POS")) -> ()
                      n497 = local write "SAME CARD DETECTED"(TRUE ("SAME CARD DETECTED")) -> ()
                      n498 = property on="STAND" class="Bool (strict)"("Val(Sgnl)"=w625) -> ()  [unwired: 2 in, 2 out]
                      n499 = Wait (ms)(milliseconds to wait=u32 1000 ("millisecond timer value")) -> ()  [unwired: 1 out]
                      n500 = local write "CP-Dealer#3"(0.0 ("CP-Dealer#3")) -> ()
                    }
                  }
                }
                n501 = for {
                  N: 1 -> [_]
                  tunnel: w546 -> [_] mode=indexing
                  n502 = local read "CP-Dealer#1"() -> (w556:dbl)
                  n503 = local read "CP-Dealer#2"() -> (w555:dbl)
                  n504 = local read "CP-Dealer#3"() -> (w554:dbl)
                  n505 = Compound Arithmetic op=ADD(w556, w555, w554) -> (w553:dbl)
                  n506 = Greater?(x=w553, y=21.0) -> (0:w551:bool)
                  n507 = case shown="False" w551 {
                    frame False {
                      w569 = 11.0 ("y")
                      w563 = 1.0 ("y")
                      n508 = local read "CP-Dealer#2"() -> (w562:dbl)
                      n509 = local read "CP-Dealer#1"() -> (w561:dbl)
                      n510 = local read "CP-Dealer#3"() -> (w573:dbl)
                      n511 = local read "Total Dealer Point"() -> (w570:dbl)
                      n512 = Equal?(x=w561, y=w563) -> (x = y?=w560:bool)
                      n513 = Equal?(x=w562, y=w563) -> (x = y?=w559:bool)
                      n514 = Equal?(x=w573, y=w563) -> (x = y?=w558:bool)
                      n515 = Add(x=w570, y=w569) -> (x+y=w572:dbl)
                      n516 = Add(x=w570, y=w569) -> (x+y=w568:dbl)
                      n517 = Greater Or Equal?(x=w568, y=17.0) -> (x >= y?=w564:bool)
                      n518 = Less Or Equal?(x=w572, y=21.0 ("x")) -> (x <= y?=w565:bool)
                      n519 = Compound Arithmetic op=OR(w560, w559, w558) -> (w557:bool)
                      n520 = Compound Arithmetic op=AND(w557, w565, w564) -> (w566:bool)
                      n521 = case shown="True" w566 {
                        selector: w566 -> [w577 _]
                        frame False {
                          n522 = local read "CP-Dealer#1"() -> (w580:dbl)
                          n523 = local read "CP-Dealer#2"() -> (w579:dbl)
                          n524 = local read "CP-Dealer#3"() -> (w578:dbl)
                          n525 = local read "Total Player Point"() -> (w575:dbl)
                          n526 = property on="STAND" class="Bool (strict)"("Val(Sgnl)"=w577) -> ()  [unwired: 2 in, 2 out]
                          n527 = Compound Arithmetic op=ADD(w580, w579, w578) -> (w576:dbl)
                          n528 = formula code="if(UP > DP && DP > 16)\nWIN = 0;\nelse if(UP < DP && DP > 16)\nWIN = 1;\nelse if(UP = DP && DP > 16)\nWIN = 2;\nelse\nWIN = 3;"("DP"=w576, "UP"=w575) -> ("WIN"=w574:dbl)
                          n529 = local write "Total Dealer Point"(w576) -> ()
                          n530 = case shown="3" w574 {
                            frame 0, Default {
                              n531 = local write "WIN"(TRUE ("WIN")) -> ()
                            }
                            frame 1 {
                              n532 = local write "LOSE"(TRUE ("LOSE")) -> ()
                            }
                            frame 2 {
                              n533 = local write "DRAW"(TRUE ("DRAW")) -> ()
                            }
                            frame 3 {
                              n534 = local write "DRAW"(FALSE ("DRAW")) -> ()
                              n535 = local write "LOSE"(FALSE ("LOSE")) -> ()
                              n536 = local write "WIN"(FALSE ("WIN")) -> ()
                            }
                          }
                        }
                        frame True {
                          n537 = local read "Total Player Point"() -> (w589:dbl)
                          n538 = local read "CP-Dealer#1"() -> (w592:dbl)
                          n539 = local read "CP-Dealer#2"() -> (w591:dbl)
                          n540 = Compound Arithmetic op=ADD(w592, w591, 11) -> (w588:dbl)
                          n541 = formula code="if(UP > DP && DP > 16)\nWIN = 0;\nelse if(UP < DP && DP > 16)\nWIN = 1;\nelse if(UP = DP && DP > 16)\nWIN = 2;\nelse\nWIN = 3;"("UP"=w589, "DP"=w588) -> ("WIN"=w587:dbl)
                          n542 = local write "Total Dealer Point"(w588) -> ()
                          n543 = case shown="2" w587 {
                            frame 0, Default {
                              n544 = local write "WIN"(TRUE ("WIN")) -> ()
                            }
                            frame 1 {
                              n545 = local write "LOSE"(TRUE ("LOSE")) -> ()
                            }
                            frame 2 {
                              n546 = local write "DRAW"(TRUE ("DRAW")) -> ()
                            }
                            frame 3 {
                              n547 = local write "DRAW"(FALSE ("DRAW")) -> ()
                              n548 = local write "LOSE"(FALSE ("LOSE")) -> ()
                              n549 = local write "WIN"(FALSE ("WIN")) -> ()
                            }
                          }
                        }
                      }
                    }
                    frame True {
                      n550 = local read "CP-Dealer#1"() -> (w603:dbl)
                      n551 = local read "CP-Dealer#2"() -> (w602:dbl)
                      n552 = local read "CP-Dealer#3"() -> (w601:dbl)
                      n553 = local write "WIN"(TRUE ("WIN")) -> ()
                      n554 = Compound Arithmetic op=ADD(w603, w602, w601) -> (w600:dbl)
                      n555 = local write "Total Dealer Point"(w600) -> ()
                    }
                  }
                }
              }
            }
          }
          frame 2 {
            n556 = local read "CP-Dealer#1"() -> (w657:dbl)
            n557 = local read "CP-Dealer#2"() -> (w656:dbl)
            n558 = local read "CP-Dealer#3"() -> (w655:dbl)
            n559 = Compound Arithmetic op=ADD(w657, w656, w655) -> (w653:dbl)
            n560 = Less?(x=w653, y=17) -> (x < y?=w652:bool)
            n561 = case shown="True" w652 {
              frame False {
              }
              frame True {
                n562 = for {
                  N: 10 -> [_]
                  tunnel: [w751] -> w661 mode=indexing
                  n563 = Random Number (0-1)() -> (number: 0 to 1=w761:dbl)
                  n564 = Wait (ms)(milliseconds to wait=u32 100) -> ()  [unwired: 1 out]
                  n565 = Multiply(x=w761, y=52) -> (x*y=w758:dbl)
                  n566 = Round To Nearest(number=w758) -> (nearest integer value=w757:dbl)
                  n567 = To Unsigned Word Integer(number=w757) -> (unsigned 16bit integer=w754:u16)
                  n568 = Greater?(x=w754, y=0.0) -> (0:w755:bool)
                  n569 = case shown="False" w755 {
                    tunnel: [w768 w771] -> w751
                    tunnel: w754 -> [w770 w771]
                    frame False {
                      n570 = Add(x=w770, y=u16 1) -> (x+y=w768:u16)
                    }
                    frame True {
                    }
                  }
                  "DealerCard#4" <- w751
                  n571 = Quotient & Remainder(x=w751, y=13) -> (x-y*floor(x/y)=w750:i32)  [unwired: 1 out]
                  n572 = Greater?(x=w750, y=10) -> (0:w749:bool)
                  n573 = case shown="False" w749 {
                    tunnel: [w763 10] -> w748
                    tunnel: w750 -> [w762 _]
                    frame False {
                      n574 = Equal To 0?(x=w762) -> (x = 0?=w764:bool)
                      n575 = case shown="True" w764 {
                        tunnel: [w765 10] -> w763
                        tunnel: w762 -> [w765 _]
                        frame False {
                        }
                        frame True {
                        }
                      }
                    }
                    frame True {
                    }
                  }
                  "CP-Dealer#4" <- w748
                }
                n576 = for {
                  N: 1 -> [_]
                  tunnel: w661 -> [w723] mode=indexing
                  tunnel: [w723] -> w659 mode=indexing
                  n577 = local read "UserCard#3"() -> (w739:u16)
                  n578 = local read "UserCard#4"() -> (w738:u16)
                  n579 = local read "UserCard#5"() -> (w737:u16)
                  n580 = local read "DealerCard#1"() -> (w736:u16)
                  n581 = local read "UserCard#1"() -> (w741:u16)
                  n582 = local read "UserCard#2"() -> (w740:u16)
                  n583 = local read "DealerCard#2"() -> (w735:u16)
                  n584 = local read "DealerCard#3"() -> (w734:u16)
                  n585 = local read "DealerCard#4"() -> (w733:u16)
                  n586 = Equal?(x=w741, y=w733) -> (x = y?=w732:bool)
                  n587 = Equal?(x=w740, y=w733) -> (x = y?=w731:bool)
                  n588 = Equal?(x=w739, y=w733) -> (x = y?=w730:bool)
                  n589 = Equal?(x=w738, y=w733) -> (x = y?=w729:bool)
                  n590 = Equal?(x=w737, y=w733) -> (x = y?=w728:bool)
                  n591 = Equal?(x=w736, y=w733) -> (x = y?=w727:bool)
                  n592 = Equal?(x=w735, y=w733) -> (x = y?=w726:bool)
                  n593 = Equal?(x=w734, y=w733) -> (x = y?=w725:bool)
                  n594 = Compound Arithmetic op=OR(w732, w731, w730, w729, w728, w727, w726, w725) -> (w724:bool)
                  n595 = case shown="False" w724 {
                    selector: w724 -> [_ w745]
                    frame False {
                      n596 = local write "STAND POS"(3.0 ("STAND POS")) -> ()
                      n597 = local write "SAME CARD DETECTED"(FALSE ("SAME CARD DETECTED")) -> ()
                    }
                    frame True {
                      n598 = property on="STAND" class="Bool (strict)"("Val(Sgnl)"=w745) -> ()  [unwired: 2 in, 2 out]
                      n599 = local write "STAND POS"(2.0 ("STAND POS")) -> ()
                      n600 = Wait (ms)(milliseconds to wait=u32 1000) -> ()  [unwired: 1 out]
                      n601 = local write "SAME CARD DETECTED"(TRUE ("SAME CARD DETECTED")) -> ()
                    }
                  }
                }
                n602 = for {
                  N: 1 -> [_]
                  tunnel: w659 -> [_] mode=indexing
                  n603 = local read "CP-Dealer#1"() -> (w669:dbl)
                  n604 = local read "CP-Dealer#2"() -> (w668:dbl)
                  n605 = local read "CP-Dealer#3"() -> (w667:dbl)
                  n606 = local read "CP-Dealer#4"() -> (w666:dbl)
                  n607 = Compound Arithmetic op=ADD(w669, w668, w667, w666) -> (w665:dbl)
                  n608 = Greater?(x=w665, y=21.0) -> (0:w663:bool)
                  n609 = case shown="False" w663 {
                    frame False {
                      w676 = 1.0 ("y")
                      w683 = 11.0 ("y")
                      n610 = local read "Total Dealer Point"() -> (w684:dbl)
                      n611 = local read "CP-Dealer#3"() -> (w677:dbl)
                      n612 = local read "CP-Dealer#1"() -> (w674:dbl)
                      n613 = local read "CP-Dealer#4"() -> (w689:dbl)
                      n614 = local read "CP-Dealer#2"() -> (w675:dbl)
                      n615 = Equal?(x=w674, y=w676) -> (x = y?=w673:bool)
                      n616 = Equal?(x=w675, y=w676) -> (x = y?=w672:bool)
                      n617 = Equal?(x=w677, y=w676) -> (x = y?=w671:bool)
                      n618 = Equal?(x=w689, y=1.0) -> (x = y?=w678:bool)
                      n619 = Add(x=w684, y=w683) -> (x+y=w687:dbl)
                      n620 = Add(x=w684, y=w683) -> (x+y=w686:dbl)
                      n621 = Greater Or Equal?(x=w687, y=17.0) -> (x >= y?=w679:bool)
                      n622 = Less Or Equal?(x=w686, y=21.0) -> (x <= y?=w680:bool)
                      n623 = Compound Arithmetic op=OR(w673, w672, w671, w678) -> (w670:bool)
                      n624 = Compound Arithmetic op=AND(w670, w680, w679) -> (w681:bool)
                      n625 = case shown="True" w681 {
                        selector: w681 -> [w697 _]
                        frame False {
                          n626 = local read "Total Player Point"() -> (w692:dbl)
                          n627 = local read "CP-Dealer#1"() -> (w696:dbl)
                          n628 = local read "CP-Dealer#2"() -> (w695:dbl)
                          n629 = local read "CP-Dealer#3"() -> (w694:dbl)
                          n630 = local read "CP-Dealer#4"() -> (w693:dbl)
                          n631 = property on="STAND" class="Bool (strict)"("Val(Sgnl)"=w697) -> ()  [unwired: 2 in, 2 out]
                          n632 = Compound Arithmetic op=ADD(w696, w695, w694, w693) -> (w691:dbl)
                          n633 = formula code="if(UP > DP && DP > 16)\nWIN = 0;\nelse if(UP < DP && DP >16)\nWIN = 1;\nelse if(UP == DP && DP >16)\nWIN = 2;\nelse\nWIN = 3;"("DP"=w691, "UP"=w692) -> ("WIN"=w690:dbl)
                          n634 = local write "Total Dealer Point"(w691) -> ()
                          n635 = case shown="1" w690 {
                            frame 0, Default {
                              n636 = local write "WIN"(TRUE ("WIN")) -> ()
                            }
                            frame 1 {
                              n637 = local write "LOSE"(TRUE ("LOSE")) -> ()
                            }
                            frame 2 {
                              n638 = local write "DRAW"(TRUE ("DRAW")) -> ()
                            }
                            frame 3 {
                              n639 = local write "DRAW"(FALSE ("DRAW")) -> ()
                              n640 = local write "LOSE"(FALSE ("LOSE")) -> ()
                              n641 = local write "WIN"(FALSE ("WIN")) -> ()
                            }
                          }
                        }
                        frame True {
                          n642 = local read "Total Player Point"() -> (w705:dbl)
                          n643 = local read "CP-Dealer#1"() -> (w707:dbl)
                          n644 = local read "CP-Dealer#2"() -> (w708:dbl)
                          n645 = local read "CP-Dealer#3"() -> (w709:dbl)
                          n646 = Compound Arithmetic op=ADD(w707, w708, w709, 11) -> (w706:dbl)
                          n647 = formula code="if(UP > DP && DP > 16)\nWIN = 0;\nelse if (UP < DP && DP > 16)\nWIN = 1;\nelse if (UP == DP && DP > 16)\nWIN = 2;\nelse\nWIN = 3;"("DP"=w706, "UP"=w705) -> ("WIN"=w704:dbl)
                          n648 = local write "Total Dealer Point"(w706) -> ()
                          n649 = case shown="0, Default" w704 {
                            frame 0, Default {
                              n650 = local write "WIN"(TRUE ("WIN")) -> ()
                            }
                            frame 1 {
                              n651 = local write "LOSE"(TRUE ("LOSE")) -> ()
                            }
                            frame 2 {
                              n652 = local write "DRAW"(TRUE ("DRAW")) -> ()
                            }
                            frame 3 {
                              n653 = local write "DRAW"(FALSE ("DRAW")) -> ()
                              n654 = local write "WIN"(FALSE ("WIN")) -> ()
                              n655 = local write "LOSE"(FALSE ("LOSE")) -> ()
                            }
                          }
                        }
                      }
                    }
                    frame True {
                      n656 = local read "CP-Dealer#4"() -> (w719:dbl)
                      n657 = local read "CP-Dealer#1"() -> (w722:dbl)
                      n658 = local read "CP-Dealer#2"() -> (w721:dbl)
                      n659 = local read "CP-Dealer#3"() -> (w720:dbl)
                      n660 = local write "WIN"(TRUE ("WIN")) -> ()
                      n661 = Compound Arithmetic op=ADD(w722, w721, w720, w719) -> (w718:dbl)
                      n662 = local write "Total Dealer Point"(w718) -> ()
                    }
                  }
                }
              }
            }
          }
          frame 3 {
            n663 = local read "CP-Dealer#1"() -> (w778:dbl)
            n664 = local read "CP-Dealer#2"() -> (w777:dbl)
            n665 = local read "CP-Dealer#3"() -> (w776:dbl)
            n666 = local read "CP-Dealer#4"() -> (w775:dbl)
            n667 = Compound Arithmetic op=ADD(w778, w777, w776, w775) -> (w774:dbl)
            n668 = Less?(x=w774, y=17) -> (x < y?=w772:bool)
            n669 = case shown="True" w772 {
              frame False {
              }
              frame True {
                n670 = for {
                  N: 10 -> [_]
                  tunnel: [w880] -> w781 mode=indexing
                  n671 = Random Number (0-1)() -> (number: 0 to 1=w890:dbl)
                  n672 = Wait (ms)(milliseconds to wait=u32 100) -> ()  [unwired: 1 out]
                  n673 = Multiply(x=w890, y=52) -> (x*y=w887:dbl)
                  n674 = Round To Nearest(number=w887) -> (nearest integer value=w886:dbl)
                  n675 = To Unsigned Word Integer(number=w886) -> (unsigned 16bit integer=w883:u16)
                  n676 = Greater?(x=w883, y=0.0) -> (0:w884:bool)
                  n677 = case shown="False" w884 {
                    tunnel: [w897 w900] -> w880
                    tunnel: w883 -> [w899 w900]
                    frame False {
                      n678 = Add(x=w899, y=u16 1) -> (x+y=w897:u16)
                    }
                    frame True {
                    }
                  }
                  "DealerCard#5" <- w880
                  n679 = Quotient & Remainder(x=w880, y=13) -> (x-y*floor(x/y)=w879:i32)  [unwired: 1 out]
                  n680 = Greater?(x=w879, y=10) -> (0:w878:bool)
                  n681 = case shown="False" w878 {
                    tunnel: [w892 10] -> w877
                    tunnel: w879 -> [w891 _]
                    frame False {
                      n682 = Equal To 0?(x=w891) -> (x = 0?=w893:bool)
                      n683 = case shown="True" w893 {
                        tunnel: [w894 10] -> w892
                        tunnel: w891 -> [w894 _]
                        frame False {
                        }
                        frame True {
                        }
                      }
                    }
                    frame True {
                    }
                  }
                  "CP-Dealer#5" <- w877
                }
                n684 = for {
                  N: 1 -> [_]
                  tunnel: w781 -> [w849] mode=indexing
                  tunnel: [w849] -> w780 mode=indexing
                  n685 = local read "DealerCard#1"() -> (w864:u16)
                  n686 = local read "DealerCard#2"() -> (w863:u16)
                  n687 = local read "DealerCard#3"() -> (w862:u16)
                  n688 = local read "DealerCard#4"() -> (w861:u16)
                  n689 = local read "DealerCard#5"() -> (w860:u16)
                  n690 = local read "UserCard#1"() -> (w869:u16)
                  n691 = local read "UserCard#2"() -> (w868:u16)
                  n692 = local read "UserCard#3"() -> (w867:u16)
                  n693 = local read "UserCard#4"() -> (w866:u16)
                  n694 = local read "UserCard#5"() -> (w865:u16)
                  n695 = Equal?(x=w869, y=w860) -> (x = y?=w859:bool)
                  n696 = Equal?(x=w868, y=w860) -> (x = y?=w858:bool)
                  n697 = Equal?(x=w867, y=w860) -> (x = y?=w857:bool)
                  n698 = Equal?(x=w866, y=w860) -> (x = y?=w856:bool)
                  n699 = Equal?(x=w865, y=w860) -> (x = y?=w855:bool)
                  n700 = Equal?(x=w864, y=w860) -> (x = y?=w854:bool)
                  n701 = Equal?(x=w863, y=w860) -> (x = y?=w853:bool)
                  n702 = Equal?(x=w862, y=w860) -> (x = y?=w852:bool)
                  n703 = Equal?(x=w861, y=w860) -> (x = y?=w851:bool)
                  n704 = Compound Arithmetic op=OR(w859, w858, w857, w856, w855, w854, w853, w852, w851) -> (w850:bool)
                  n705 = case shown="True" w850 {
                    selector: w850 -> [w870 w875]
                    frame False {
                      n706 = local write "STAND POS"(4.0 ("STAND POS")) -> ()
                      n707 = local write "SAME CARD DETECTED"(FALSE ("SAME CARD DETECTED")) -> ()
                      n708 = property on="STAND" class="Bool (strict)"("Val(Sgnl)"=w870) -> ()  [unwired: 2 in, 2 out]
                    }
                    frame True {
                      n709 = property on="STAND" class="Bool (strict)"("Val(Sgnl)"=w875) -> ()  [unwired: 2 in, 2 out]
                      n710 = local write "STAND POS"(3.0 ("STAND POS")) -> ()
                      n711 = local write "SAME CARD DETECTED"(TRUE ("SAME CARD DETECTED")) -> ()
                      n712 = Wait (ms)(milliseconds to wait=u32 1000) -> ()  [unwired: 1 out]
                    }
                  }
                }
                n713 = for {
                  N: 1 -> [_]
                  tunnel: w780 -> [_] mode=indexing
                  n714 = local read "CP-Dealer#1"() -> (w791:dbl)
                  n715 = local read "CP-Dealer#2"() -> (w790:dbl)
                  n716 = local read "CP-Dealer#3"() -> (w789:dbl)
                  n717 = local read "CP-Dealer#4"() -> (w788:dbl)
                  n718 = local read "CP-Dealer#5"() -> (w787:dbl)
                  n719 = Compound Arithmetic op=ADD(w791, w790, w789, w788, w787) -> (w786:dbl)
                  n720 = Greater?(x=w786, y=21.0) -> (0:w784:bool)
                  n721 = case shown="False" w784 {
                    frame False {
                      w795 = 1.0 ("x")
                      w808 = 11
                      n722 = local read "CP-Dealer#1"() -> (w792:dbl)
                      n723 = local read "CP-Dealer#2"() -> (w793:dbl)
                      n724 = local read "Total Dealer Point"() -> (w809:dbl)
                      n725 = local read "CP-Dealer#5"() -> (w813:dbl)
                      n726 = local read "CP-Dealer#3"() -> (w794:dbl)
                      n727 = local read "CP-Dealer#4"() -> (w800:dbl)
                      n728 = Equal?(x=w813, y=1.0) -> (x = y?=w801:bool)
                      n729 = Equal?(x=w792, y=w795) -> (x = y?=w796:bool)
                      n730 = Equal?(x=w793, y=w795) -> (x = y?=w797:bool)
                      n731 = Equal?(x=w794, y=w795) -> (x = y?=w798:bool)
                      n732 = Equal?(x=w795, y=w800) -> (x = y?=w799:bool)
                      n733 = Add(x=w809, y=w808) -> (x+y=w806:dbl)
                      n734 = Add(x=w809, y=w808) -> (x+y=w811:dbl)
                      n735 = Greater Or Equal?(x=w806, y=17.0 ("x")) -> (x >= y?=w804:bool)
                      n736 = Less Or Equal?(x=w811, y=21.0) -> (x <= y?=w805:bool)
                      n737 = Compound Arithmetic op=OR(w796, w797, w798, w799, w801) -> (w802:bool)
                      n738 = Compound Arithmetic op=AND(w802, w805, w804) -> (w803:bool)
                      n739 = case shown="True" w803 {
                        frame False {
                          n740 = local read "CP-Dealer#1"() -> (w821:dbl)
                          n741 = local read "CP-Dealer#2"() -> (w820:dbl)
                          n742 = local read "CP-Dealer#3"() -> (w819:dbl)
                          n743 = local read "CP-Dealer#4"() -> (w818:dbl)
                          n744 = local read "CP-Dealer#5"() -> (w817:dbl)
                          n745 = local read "Total Player Point"() -> (w815:dbl)
                          n746 = Compound Arithmetic op=ADD(w821, w820, w819, w818, w817) -> (w816:dbl)
                          n747 = formula code="if(UP > DP && DP > 16)\nWIN = 0;\nelse if(UP < DP && DP > 16)\nWIN = 1;\nelse if(UP == DP && DP > 16) \nWIN = 2;\nelse\nWIN = 3;"("UP"=w815, "DP"=w816) -> ("WIN"=w814:dbl)
                          n748 = local write "Total Dealer Point"(w816) -> ()
                          n749 = case shown="3" w814 {
                            frame 0, Default {
                              n750 = local write "WIN"(TRUE ("WIN")) -> ()
                            }
                            frame 1 {
                              n751 = local write "LOSE"(TRUE ("LOSE")) -> ()
                            }
                            frame 2 {
                              n752 = local write "DRAW"(TRUE ("DRAW")) -> ()
                            }
                            frame 3 {
                              n753 = local write "DRAW"(FALSE ("DRAW")) -> ()
                              n754 = local write "LOSE"(FALSE ("LOSE")) -> ()
                              n755 = local write "WIN"(FALSE ("WIN")) -> ()
                            }
                          }
                        }
                        frame True {
                          n756 = local read "Total Player Point"() -> (w829:dbl)
                          n757 = local read "CP-Dealer#2"() -> (w834:dbl)
                          n758 = local read "CP-Dealer#1"() -> (w835:dbl)
                          n759 = local read "CP-Dealer#3"() -> (w833:dbl)
                          n760 = local read "CP-Dealer#4"() -> (w832:dbl)
                          n761 = Compound Arithmetic op=ADD(w835, w834, w833, w832, 11) -> (w830:dbl)
                          n762 = formula code="if(UP>DP && DP > 16)\nWIN = 0;\nelse if(UP < DP && DP > 16)\nWIN = 1;\nelse if(UP == DP && DP > 16)\nWIN = 2;\nelse\nWIN = 3;"("UP"=w829, "DP"=w830) -> ("WIN"=w828:dbl)
                          n763 = local write "Total Dealer Point"(w830) -> ()
                          n764 = case shown="3" w828 {
                            frame 0, Default {
                              n765 = local write "WIN"(TRUE ("WIN")) -> ()
                            }
                            frame 1 {
                              n766 = local write "LOSE"(TRUE ("LOSE")) -> ()
                            }
                            frame 2 {
                              n767 = local write "DRAW"(TRUE ("DRAW")) -> ()
                            }
                            frame 3 {
                              n768 = local write "DRAW"(FALSE ("DRAW")) -> ()
                              n769 = local write "LOSE"(FALSE ("LOSE")) -> ()
                              n770 = local write "WIN"(FALSE ("WIN")) -> ()
                            }
                          }
                        }
                      }
                    }
                    frame True {
                      n771 = local read "CP-Dealer#2"() -> (w847:dbl)
                      n772 = local read "CP-Dealer#5"() -> (w844:dbl)
                      n773 = local read "CP-Dealer#1"() -> (w848:dbl)
                      n774 = local read "CP-Dealer#3"() -> (w846:dbl)
                      n775 = local read "CP-Dealer#4"() -> (w845:dbl)
                      n776 = local write "WIN"(TRUE ("WIN")) -> ()
                      n777 = Compound Arithmetic op=ADD(w848, w847, w846, w845, w844) -> (w843:dbl)
                      n778 = local write "Total Dealer Point"(w843) -> ()
                    }
                  }
                }
              }
            }
          }
        }
      }
      event "RESTART GAME": Value Change {
        n779 = event-data() -> ()  [unwired: 1 in, 4 out]
        n780 = control-ref of="This VI"() -> (w903:refnum<vi>)
        n781 = invoke class="VI" method="Default Vals.Reinit All"(reference=w903) -> (reference out=w902:refnum<vi>, error out=w901:errorcluster)  [unwired: 2 in, 1 out]
        n782 = Close Reference(reference=w902, error in (no error)=w901) -> ()  [unwired: 1 out]
      }
      event "EMERGENCY STOP": Value Change {
        n783 = event-data() -> ()  [unwired: 1 in, 1 out]
      }
    }
    "Numeric" <- w2
  }
